vi "SWT.vi"(0 "System no.":i32=1 min=1 max=4 step=1, 2 "Axis":string, 3 "Max. n values":i32=64, 4 "No.of digits":i16=3, 5 "error in":errorcluster, 6 "Ao,...,An-1":dbl[](array[numeric])=[0.001, 0.002, 0.003, 0.004, 0.005, 0.006, 0.007, 0.008, 0.009, 0.01] format="%.6f") -> (14 "Successful?":bool, 19 "error out":errorcluster)   [LabVIEW 2026]
doc: "This VI defines a waveform for one axis. Data points are transferred point by point. Max. n values is the maximum number of points that can be transferred. No. of digits is the number of digits after the decimal point in the data point value(s) that will be sent. Please refer to the system manual for units and restrictions. \n\nE-816: Max. n values = 64"
panel:
  # "This vi defines a waveform for one axis. Data points are transferred point\nby point. Max. n values is the maximum number of points that can be\ntransferred. Please refer to the system manual for units and restrictions."
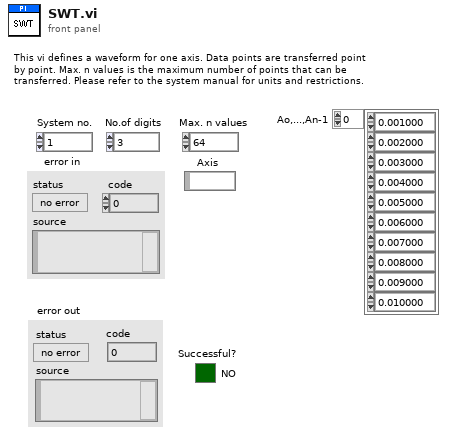
[diagram p1: front panel]
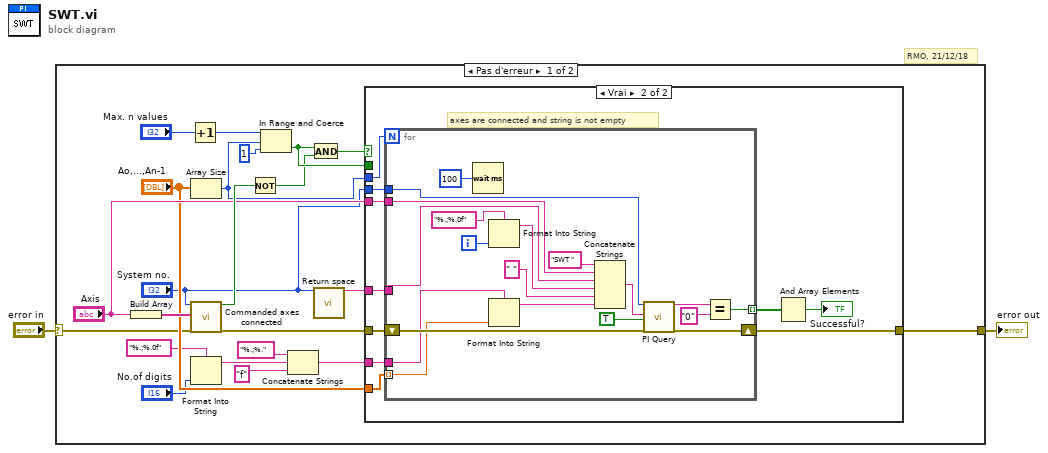
[diagram p0: block diagram]
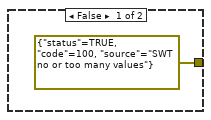
[diagram p3: hidden frame]
diagram:
  # "RMO, 21/12/18"
  n1 = case shown="Pas d'erreur" "error in" {
    selector: "error in" -> [w3 w59]
    tunnel: [w24 w59] -> w2
    frame No Error {
      n2 = Build Array("Axis") -> (w15:string[])
      n3 = Increment(x="Max. n values") -> (x+1=w20:i32)
      n4 = Array Size(array="Ao,...,An-1") -> (size(s)=w13:i32)
      n5 = call "Commanded axes connected.vi"("System no."="System no.", "Commanded axes"=w15, "error in"=w3) -> ("Controller error"=w18:bool, "error out"=w23:errorcluster)  [unwired: 1 in, 14 out]
      n6 = Format Into String(format string="%.;%.0f" ("Format String"), "No.of digits") -> (resulting string=w6:string)  [unwired: 2 in, 1 out]
      n7 = Not(x=w18) -> (.not. x?=w17:bool)
      n8 = In Range and Coerce(upper limit=w20, x=w13, lower limit=1 ("lo")) -> (In Range?=w19:bool)  [unwired: 1 out]
      n9 = Concatenate Strings("%.;%." ("Format String"), w6, "f" ("Format String")) -> (w5:string)
      n10 = And(x=w19, y=w17) -> (x .and. y?=w16:bool)
      n11 = call "Return space.vi"("System no."="System no.") -> ("String out"=w10:string)  [unwired: 1 in, 17 out]
      n12 = case shown="Vrai" w16 {
        tunnel: [w27 w31] -> w24
        tunnel: w23 -> [w25 w38]
        tunnel: "System no." -> [_ w39]
        tunnel: w19 -> [w26 _]
        tunnel: "Axis" -> [_ w37]
        tunnel: w13 -> [_ w36]
        tunnel: "Ao,...,An-1" -> [_ w35]
        tunnel: w5 -> [_ w34]
        tunnel: w10 -> [_ w30]
        frame False {
          # "substring empty or axis not connected"
          n13 = case shown="Vrai" w26 {
            tunnel: [errorcluster {"status"=TRUE, "code"=100, "source"="SWT no or too many values"} ("error out") w29] -> w27
            tunnel: w25 -> [_ w29]
            frame False {
            }
            frame True {
            }
          }
        }
        frame True {
          # "axes are connected and string is not empty"
          n14 = for {
            N: w36 -> [_]
            tunnel: w39 -> [w49]
            shift-right: [w40] -> w31
            shift-left: w38 -> [w56]
            tunnel: w37 -> [w55]
            tunnel: w35 -> [w52] mode=indexing
            tunnel: w34 -> [w51]
            tunnel: [w48] -> w33 mode=indexing
            tunnel: w30 -> [w42]
            i -> [w54]
            n15 = Wait (ms)(milliseconds to wait=u32 100) -> ()  [unwired: 1 out]
            n16 = Format Into String(format string="%.;%.0f" ("Format String"), w54) -> (resulting string=w43:string)  [unwired: 2 in, 1 out]
            n17 = Format Into String(format string=w51, w52) -> (resulting string=w45:string)  [unwired: 2 in, 1 out]
            n18 = Concatenate Strings("SWT ", w55, w42, w43, " " ("Substring"), w45) -> (w47:string)
            n19 = call "PI Query.vi"("System no."=w49, "String to send"=w47, "Attach termination char.?"=TRUE ("Attach Linefeed?"), "error in"=w56) -> ("String read"=w41:string, "error out"=w40:errorcluster)  [unwired: 3 in, 11 out]
            n20 = Equal?(x=w41, y="0") -> (x = y?=w48:bool)
          }
          n21 = And Array Elements(Boolean array=w33) -> (logical AND=→"Successful?":bool)
        }
      }
    }
    frame Error {
    }
  }
  "error out" <- w2
